vi "Clear maps and sessions.vi"(8 "error in":errorcluster, 11 "References":T1) -> (0 "error out":errorcluster)   [LabVIEW 2025, in "CAN-LIN Raw Bus Capture UI.lvlib"]
uses:
  CAN-LIN Raw Bus Capture UI.lvlib
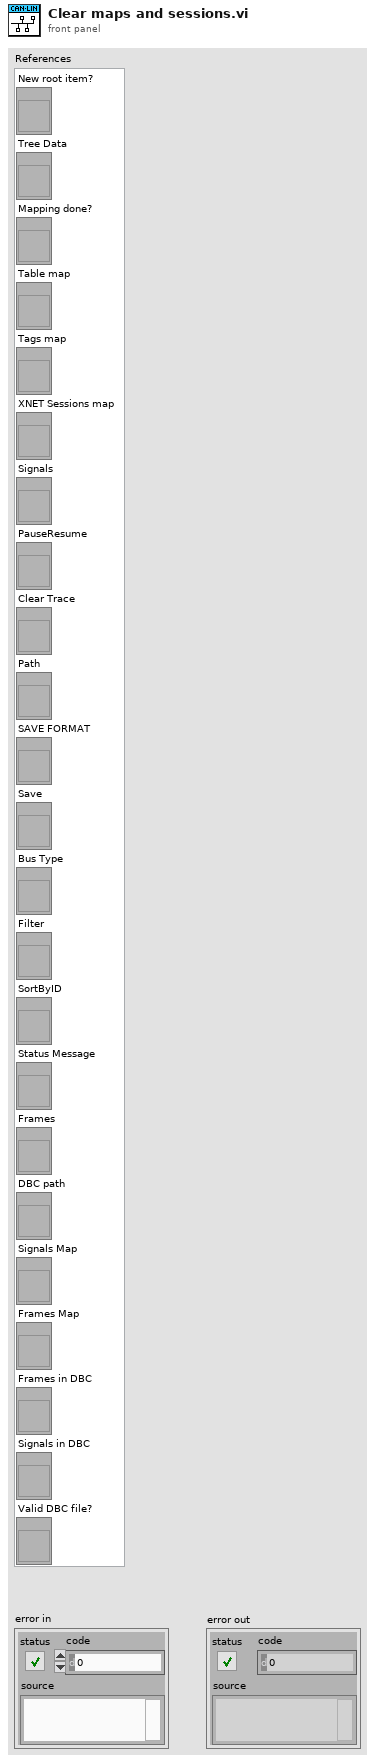
[diagram p1: front panel]
types:
  T1 = cluster{"New root item?":refnum<vi>, "Tree Data":refnum<vi>, "Mapping done?":refnum<vi>, "Table map":refnum<vi>, "Tags map":refnum<vi>, "XNET Sessions map":refnum<vi>, "Signals":refnum<vi>, "PauseResume":refnum<vi>, "Clear Trace":refnum<vi>, "Path":refnum<vi>, "SAVE FORMAT":refnum<vi>, "Save":refnum<vi>, "Bus Type":refnum<vi>, "Filter":refnum<vi>, "SortByID":refnum<vi>, "Status Message":refnum<vi>, "Frames":refnum<vi>, "DBC path":refnum<vi>, "Signals Map":refnum<vi>, "Frames Map":refnum<vi>, "Frames in DBC":refnum<vi>, "Signals in DBC":refnum<vi>, "Valid DBC file?":refnum<vi>}
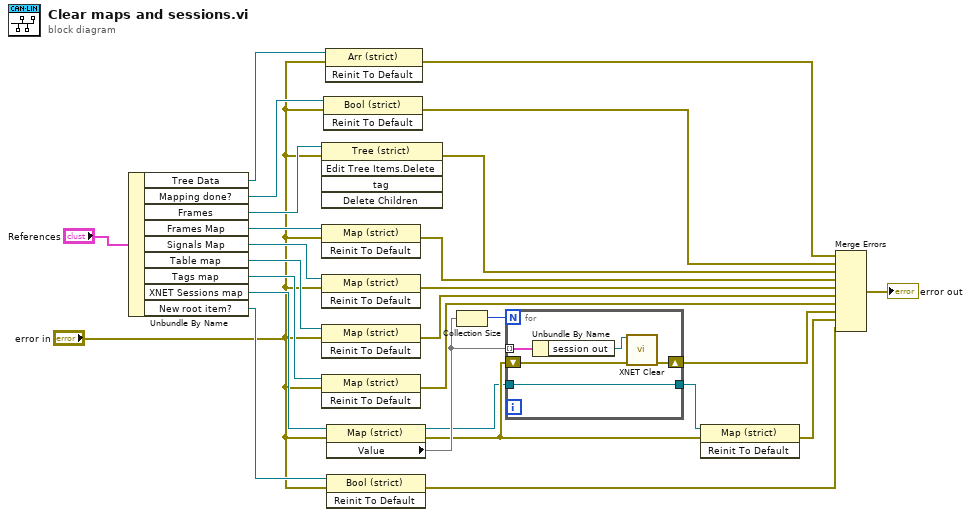
[diagram p0: block diagram]
diagram:
  n1 = Unbundle By Name("References") -> ("Tree Data"=w6:refnum<vi>, "Mapping done?"=w8:refnum<vi>, "Frames"=w22:refnum<vi>, "Frames Map"=w21:refnum<vi>, "Signals Map"=w20:refnum<vi>, "Table map"=w19:refnum<vi>, "Tags map"=w18:refnum<vi>, "XNET Sessions map"=w16:refnum<vi>, "New root item?"=w3:refnum<vi>)
  n2 = invoke on="Invoke Node" class="Tree (strict)" method="Edit Tree Items.Delete"(reference=w22, error in="error in") -> (error out=w24:errorcluster)  [unwired: 3 in, 4 out]
  n3 = invoke class="Map (strict)" method="Reinit To Default"(reference=w21, error in="error in") -> (error out=w23:errorcluster)  [unwired: 1 in, 2 out]
  n4 = invoke class="Map (strict)" method="Reinit To Default"(reference=w20, error in="error in") -> (error out=w11:errorcluster)  [unwired: 1 in, 2 out]
  n5 = invoke class="Map (strict)" method="Reinit To Default"(reference=w19, error in="error in") -> (error out=w12:errorcluster)  [unwired: 1 in, 2 out]
  n6 = invoke class="Map (strict)" method="Reinit To Default"(reference=w18, error in="error in") -> (error out=w17:errorcluster)  [unwired: 1 in, 2 out]
  n7 = invoke class="Bool (strict)" method="Reinit To Default"(reference=w8, error in="error in") -> (error out=w7:errorcluster)  [unwired: 1 in, 2 out]
  n8 = invoke class="Arr (strict)" method="Reinit To Default"(reference=w6, error in="error in") -> (error out=w5:errorcluster)  [unwired: 1 in, 2 out]
  n9 = property class="Map (strict)"(reference=w16, error in="error in") -> (reference out=w9:refnum<vi>, error out=w15:errorcluster, "Value"=w26:map{u32, refnum<k21>})
  n10 = invoke class="Bool (strict)" method="Reinit To Default"(reference=w3, error in="error in") -> (error out=w1:errorcluster)  [unwired: 1 in, 2 out]
  n11 = Collection Size(1:w26) -> (0:w27:i32)
  n12 = for {
    N: w27 -> [_]
    tunnel: w26 -> [w32] mode=indexing
    shift-right: [w29] -> w13
    shift-left: w15 -> [w30]
    tunnel: [w28] -> w10
    tunnel: w9 -> [w28]
    n13 = Unbundle By Name(w32) -> ("session out"=w31:refnum<k21>)
    n14 = call <vilib>:"XNET Clear.vi"("session in"=w31, "error in (no error)"=w30) -> ("error out"=w29:errorcluster)  [unwired: 13 in]
  }
  n15 = invoke class="Map (strict)" method="Reinit To Default"(reference=w10, error in=w15) -> (error out=w14:errorcluster)  [unwired: 1 in, 2 out]
  n16 = Merge Errors(w5, w7, w24, w23, w11, w12, w17, w13, w14, w1) -> (→"error out":errorcluster)
